vi "ex_CheckAllT0DtEqualWfm.vi"(1 "Signals":waveform(dbl)[](array[waveform])) -> (0 "All dt and t0 equal?":bool)   [LabVIEW 2017]
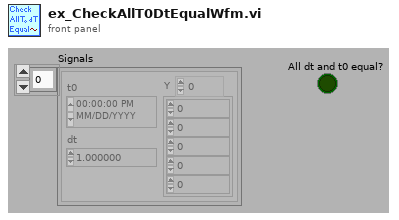
[diagram p1: front panel]
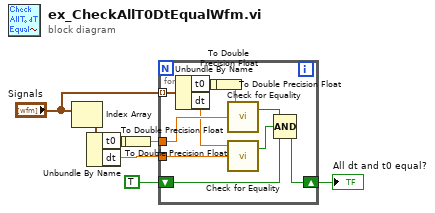
[diagram p0: block diagram]
diagram:
  n1 = Index Array(array="Signals") -> (element=w3:waveform(dbl))  [unwired: 1 in]
  n2 = Unbundle By Name(w3) -> ("t0"=w1:timestamp, "dt"=w6:dbl)
  n3 = To Double Precision Float(number=w1) -> (double precision float=w2:dbl)
  n4 = To Double Precision Float(number=w2) -> (double precision float=w5:dbl)
  n5 = for {
    tunnel: "Signals" -> [w19] mode=indexing
    shift-right: [w14] -> w7
    shift-left: TRUE -> [w13]
    tunnel: w5 -> [w17]
    tunnel: w6 -> [w15]
    n6 = Unbundle By Name(w19) -> ("t0"=w9:timestamp, "dt"=w16:dbl)
    n7 = To Double Precision Float(number=w9) -> (double precision float=w10:dbl)
    n8 = To Double Precision Float(number=w10) -> (double precision float=w18:dbl)
    n9 = call <vilib>:"Check for Equality.vi"("n2"=w17, "n1"=w18) -> ("equal?"=w11:bool)  [unwired: 2 out]
    n10 = call <vilib>:"Check for Equality.vi"("n2"=w15, "n1"=w16) -> ("equal?"=w12:bool)  [unwired: 2 out]
    n11 = Compound Arithmetic op=AND(w11, w12, w13) -> (w14:bool)
  }
  "All dt and t0 equal?" <- w7
